vi "抽样2.vi"(7 "时间标识":timestamp, 8 "采样数":dbl, 10 "采集数据":dbl[][](array[numeric]), 11 "采样率":i32[](array[numeric])=[400000, 400000, 400000, 400000, 400000, 400000, 400000, 400000]) -> (3 "6133":T1, 5 "抽样耗时ms":u32)   [LabVIEW 2014]
panel:
  out "抽样耗时s":dbl
  out "毫秒计时值":u32
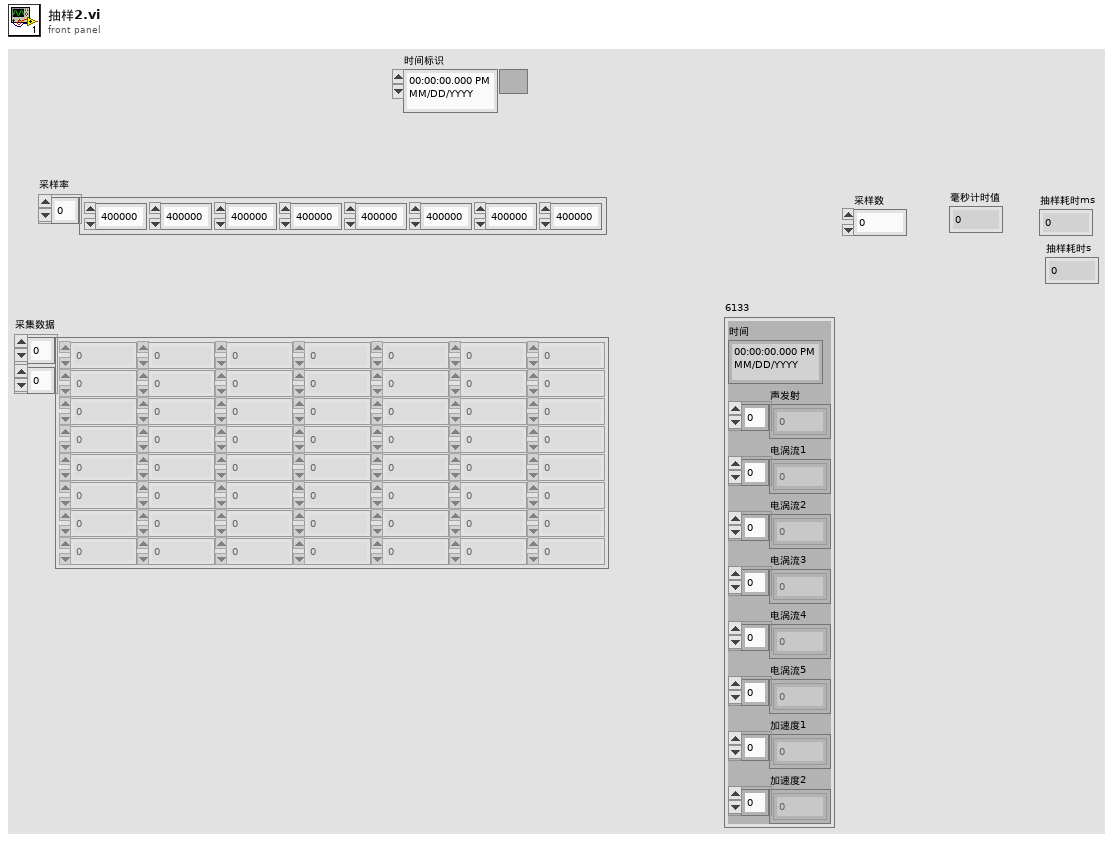
[diagram p1: front panel]
types:
  T1 = cluster{"时间":timestamp, "声发射":sgl[], "电涡流1":sgl[], "电涡流2":sgl[], "电涡流3":sgl[], "电涡流4":sgl[], "电涡流5":sgl[], "加速度1":sgl[], "加速度2":sgl[]}
  T2 = cluster{"时间标识":timestamp, dbl[], dbl[], dbl[], dbl[], dbl[], dbl[], dbl[], dbl[]}
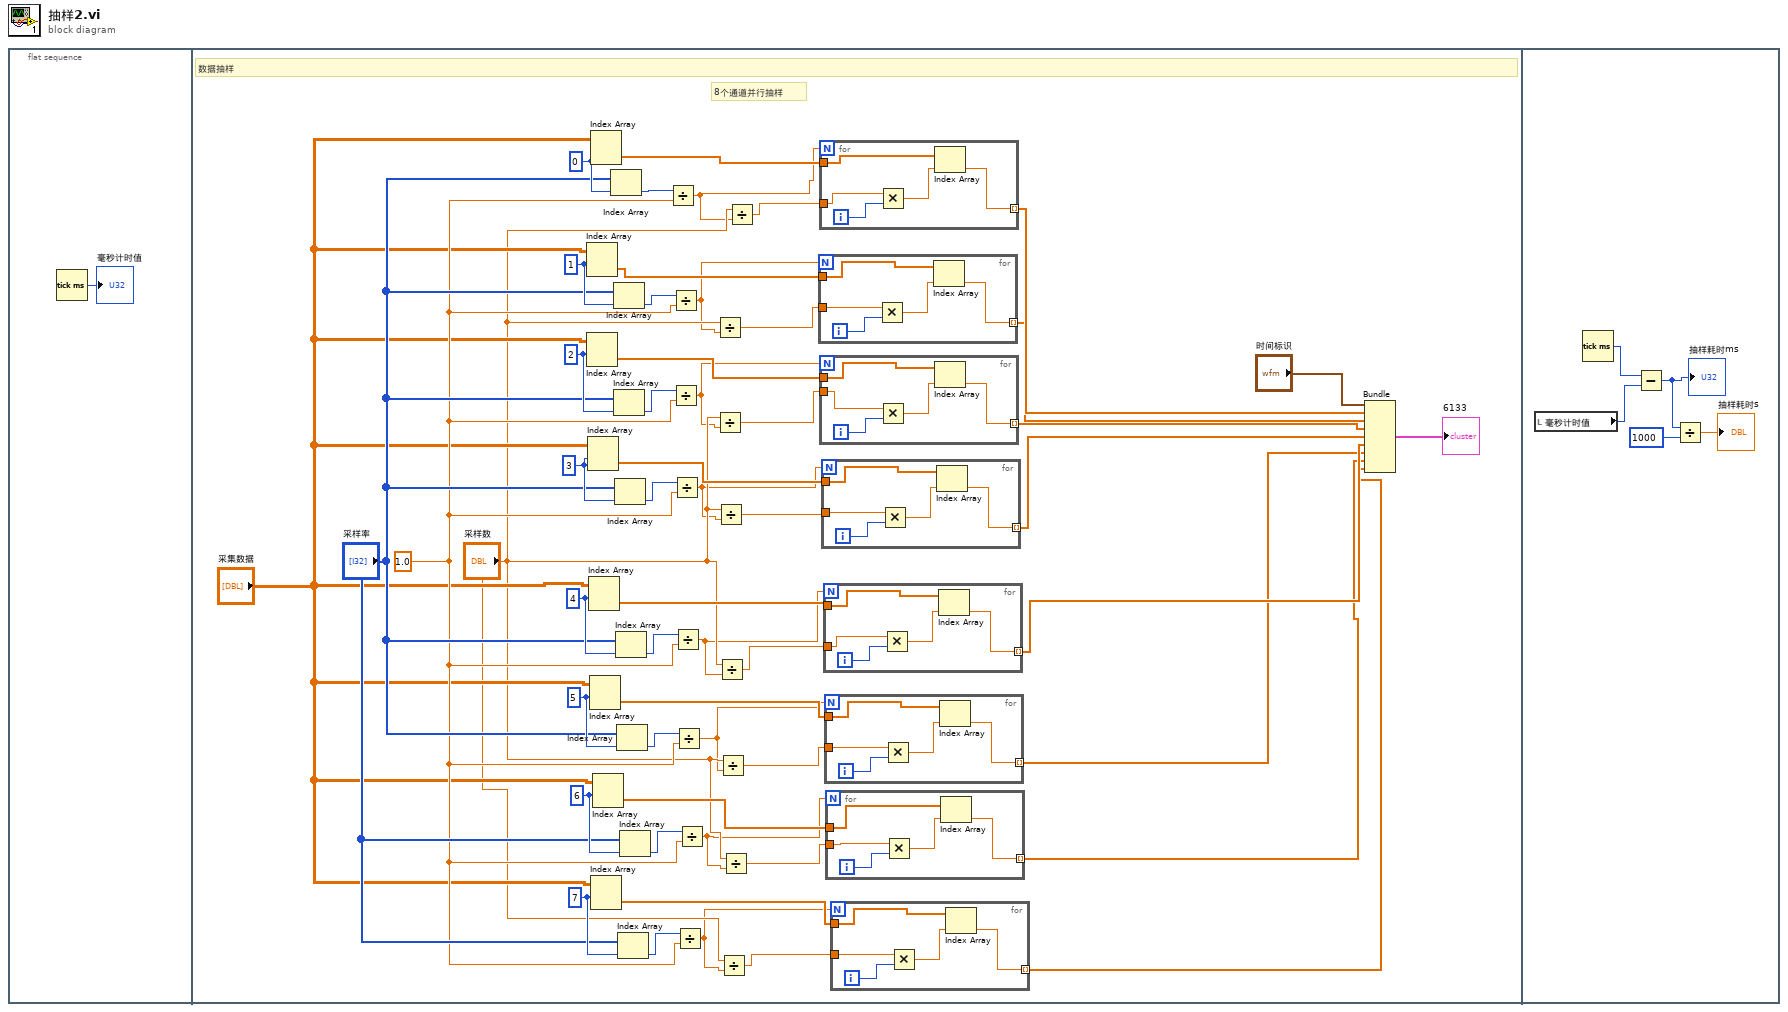
[diagram p0: block diagram]
diagram:
  n1 = flat-sequence "平铺式顺序结构" {
    frame #0 {
      n2 = Tick Count (ms)() -> (millisecond timer value=→"毫秒计时值":u32)
    }
    frame #1 {
      w38 = 1.0 ("读取次数")
      w41 = 7 ("索引")
      w43 = 6 ("索引")
      w45 = 5 ("索引")
      w47 = 4 ("索引")
      w49 = 3 ("索引")
      w51 = 2 ("索引")
      w53 = 1 ("索引")
      w55 = 0 ("索引")
      # "8个通道并行抽样"
      # "数据抽样"
      n3 = Index Array(array="采集数据", index (row)=w53) -> (element=w30:dbl[])  [unwired: 1 in]
      n4 = Index Array(array="采集数据", index (row)=w51) -> (element=w31:dbl[])  [unwired: 1 in]
      n5 = Index Array(array="采集数据", index (row)=w49) -> (element=w32:dbl[])  [unwired: 1 in]
      n6 = Index Array(array="采集数据", index (row)=w47) -> (element=w33:dbl[])  [unwired: 1 in]
      n7 = Index Array(array="采集数据", index (row)=w45) -> (element=w34:dbl[])  [unwired: 1 in]
      n8 = Index Array(array="采集数据", index (row)=w55) -> (element=w29:dbl[])  [unwired: 1 in]
      n9 = Index Array(array="采集数据", index (row)=w41) -> (element=w36:dbl[])  [unwired: 1 in]
      n10 = Index Array(array="采集数据", index (row)=w43) -> (element=w35:dbl[])  [unwired: 1 in]
      n11 = Index Array(array="采样率", index=w55) -> (element=w54:i32)
      n12 = Index Array(array="采样率", index=w53) -> (element=w52:i32)
      n13 = Index Array(array="采样率", index=w51) -> (element=w50:i32)
      n14 = Index Array(array="采样率", index=w49) -> (element=w48:i32)
      n15 = Index Array(array="采样率", index=w47) -> (element=w46:i32)
      n16 = Index Array(array="采样率", index=w45) -> (element=w44:i32)
      n17 = Index Array(array="采样率", index=w41) -> (element=w40:i32)
      n18 = Index Array(array="采样率", index=w43) -> (element=w42:i32)
      n19 = Divide(x=w54, y=w38) -> (x/y=w24:dbl)
      n20 = Divide(x=w52, y=w38) -> (x/y=w22:dbl)
      n21 = Divide(x=w50, y=w38) -> (x/y=w21:dbl)
      n22 = Divide(x=w48, y=w38) -> (x/y=w19:dbl)
      n23 = Divide(x=w46, y=w38) -> (x/y=w27:dbl)
      n24 = Divide(x=w44, y=w38) -> (x/y=w16:dbl)
      n25 = Divide(x=w40, y=w38) -> (x/y=w13:dbl)
      n26 = Divide(x=w42, y=w38) -> (x/y=w14:dbl)
      n27 = Divide(x="采样数", y=w22) -> (x/y=w23:dbl)
      n28 = Divide(x="采样数", y=w21) -> (x/y=w20:dbl)
      n29 = Divide(x="采样数", y=w19) -> (x/y=w18:dbl)
      n30 = Divide(x="采样数", y=w27) -> (x/y=w26:dbl)
      n31 = Divide(x="采样数", y=w16) -> (x/y=w17:dbl)
      n32 = Divide(x="采样数", y=w13) -> (x/y=w12:dbl)
      n33 = Divide(x="采样数", y=w14) -> (x/y=w15:dbl)
      n34 = Divide(x="采样数", y=w24) -> (x/y=w25:dbl)
      n35 = for {
        N: w22 -> [_]
        tunnel: [w65] -> w10 mode=indexing
        tunnel: w30 -> [w62]
        tunnel: w23 -> [w61]
        i -> [w64]
        n36 = Multiply(x=w61, y=w64) -> (x*y=w63:dbl)
        n37 = Index Array(array=w62, index=w63) -> (element=w65:dbl)
      }
      n38 = for {
        N: w24 -> [_]
        tunnel: [w60] -> w11 mode=indexing
        tunnel: w29 -> [w57]
        tunnel: w25 -> [w56]
        i -> [w59]
        n39 = Multiply(x=w56, y=w59) -> (x*y=w58:dbl)
        n40 = Index Array(array=w57, index=w58) -> (element=w60:dbl)
      }
      n41 = for {
        N: w21 -> [_]
        tunnel: [w70] -> w8 mode=indexing
        tunnel: w31 -> [w67]
        tunnel: w20 -> [w66]
        i -> [w69]
        n42 = Multiply(x=w66, y=w69) -> (x*y=w68:dbl)
        n43 = Index Array(array=w67, index=w68) -> (element=w70:dbl)
      }
      n44 = for {
        N: w19 -> [_]
        tunnel: [w75] -> w7 mode=indexing
        tunnel: w32 -> [w72]
        tunnel: w18 -> [w71]
        i -> [w74]
        n45 = Multiply(x=w71, y=w74) -> (x*y=w73:dbl)
        n46 = Index Array(array=w72, index=w73) -> (element=w75:dbl)
      }
      n47 = for {
        N: w27 -> [_]
        tunnel: [w80] -> w6 mode=indexing
        tunnel: w33 -> [w77]
        tunnel: w26 -> [w76]
        i -> [w79]
        n48 = Multiply(x=w76, y=w79) -> (x*y=w78:dbl)
        n49 = Index Array(array=w77, index=w78) -> (element=w80:dbl)
      }
      n50 = for {
        N: w16 -> [_]
        tunnel: [w85] -> w5 mode=indexing
        tunnel: w34 -> [w82]
        tunnel: w17 -> [w81]
        i -> [w84]
        n51 = Multiply(x=w81, y=w84) -> (x*y=w83:dbl)
        n52 = Index Array(array=w82, index=w83) -> (element=w85:dbl)
      }
      n53 = for {
        N: w14 -> [_]
        tunnel: [w90] -> w4 mode=indexing
        tunnel: w35 -> [w87]
        tunnel: w15 -> [w86]
        i -> [w89]
        n54 = Multiply(x=w86, y=w89) -> (x*y=w88:dbl)
        n55 = Index Array(array=w87, index=w88) -> (element=w90:dbl)
      }
      n56 = for {
        N: w13 -> [_]
        tunnel: [w95] -> w3 mode=indexing
        tunnel: w36 -> [w92]
        tunnel: w12 -> [w91]
        i -> [w94]
        n57 = Multiply(x=w91, y=w94) -> (x*y=w93:dbl)
        n58 = Index Array(array=w92, index=w93) -> (element=w95:dbl)
      }
      n59 = Bundle("时间标识"="时间标识", w11, w10, w8, w7, w6, w5, w4, w3) -> (→"6133":T2)  [unwired: 1 in]
    }
    frame #2 {
      n60 = local read "毫秒计时值"() -> (w99:u32)
      n61 = Tick Count (ms)() -> (millisecond timer value=w100:u32)
      n62 = Subtract(x=w100, y=w99) -> (x-y=w98:u32)
      "抽样耗时ms" <- w98
      n63 = Divide(x=w98, y=u32 1000) -> (x/y=→"抽样耗时s":dbl)
    }
  }
